vi "Periodic Tasks.vi"(8 "error in":errorcluster) -> ()   [LabVIEW 2018]
doc: "This VI runs in parallel to other tasks. It can contain as many user-defined periodic loops as you need. These can carry out PID or other sorts of timed response."
uses:
  <vilib>/Rock Robotics/WPI/Solenoid/WPI_SolenoidValue.ctl
  <vilib>/Rock Robotics/WPI/ThirdParty/Phoenix-LabVIEW/Motor Controller/Controls/CTRE_Phoenix_MotorControl_ControlMode.ctl
  <vilib>/Rock Robotics/WPI/Utilities/WPI_GetSetVariantRefNum.vi
  <vilib>/Rock Robotics/WPI/Solenoid/WPI_SolenoidSetEnum.vi
  <vilib>/Rock Robotics/WPI/ThirdParty/Phoenix-LabVIEW/Motor Controller/Get/CTRE_Phoenix_MotorController_GetQuadratureData.vi
  <vilib>/Rock Robotics/WPI/ThirdParty/Phoenix-LabVIEW/Pigeon IMU/CTRE_PigeonIMU_GetYPR.vi
  <vilib>/Rock Robotics/WPI/ThirdParty/Phoenix-LabVIEW/Pigeon IMU/CTRE_PigeonIMU_GetRawGyro.vi
  <vilib>/Rock Robotics/WPI/ThirdParty/Phoenix-LabVIEW/Pigeon IMU/CTRE_PigeonIMU_GetTempStateUpTime.vi
  <vilib>/Rock Robotics/Network Tables/NT Write Numeric Array.vi
  <vilib>/Rock Robotics/Network Tables/NT Read Number.vi
  <vilib>/addons/control/pid/pid.llb/PID Gain Schedule (DBL).vi
  <vilib>/addons/control/pid/pid.llb/PID (DBL).vi
  <vilib>/Rock Robotics/WPI/ThirdParty/Phoenix-LabVIEW/Pigeon IMU/CTRE_PigeonIMU_PigeonState.ctl
  <vilib>/addons/control/pid/NI_PID_pid.lvlib
panel:
  in  "M":dbl=0.0005
  out "X VISION":dbl=-0.020652084350585936
  out "tx":dbl=0.1304168701171875
  in  "Offset":dbl
  out "index out":i32
  in  "PID gain schedule":T1(array[cluster])=[{"PID gains"={"proportional gain (Kc)"=0.005, "integral time (Ti, min)"=0.0, "derivative time (Td, min)"=0.003}, "max value"=5.0}, {"PID gains"={"proportional gain (Kc)"=0.0105, "integral time (Ti, min)"=0.0, "derivative time (Td, min)"=0.003}, "max value"=8.0}, {"PID gains"={"proportional gain (Kc)"=0.024, "integral time (Ti, min)"=0.0, "derivative time (Td, min)"=0.0}, "max value"=12.0}, {"PID gains"={"proportional gain (Kc)"=0.02, "integral time (Ti, min)"=0.0, "derivative time (Td, min)"=0.0}, "max value"=18.0}, {"PID gains"={"proportional gain (Kc)"=0.01, "integral time (Ti, min)"=0.0, "derivative time (Td, min)"=0.0}, "max value"=25.0}] {"max value" format="%.2f"; "PID gains"."derivative time (Td, min)" format="%.3f"; "PID gains"."integral time (Ti, min)" format="%.3f"; "PID gains"."proportional gain (Kc)" format="%.3f"}
  out "tx":dbl=0.1304168701171875
  in  "Offset":dbl
  out "Left Drive Position":i32
  out "Right Drive Position":i32
  out "Right Drive Velocity":i32(graph)
  out "Left Drive Velocity":i32(graph)
  out "X VISION":dbl=-0.020652084350585936
  in  "X-Offset":dbl
  in  "PID gain schedule for vision":T1(array[cluster])=[{"PID gains"={"proportional gain (Kc)"=0.005, "integral time (Ti, min)"=0.0, "derivative time (Td, min)"=0.003}, "max value"=5.0}, {"PID gains"={"proportional gain (Kc)"=0.0105, "integral time (Ti, min)"=0.0, "derivative time (Td, min)"=0.003}, "max value"=8.0}, {"PID gains"={"proportional gain (Kc)"=0.024, "integral time (Ti, min)"=0.0, "derivative time (Td, min)"=0.0}, "max value"=12.0}, {"PID gains"={"proportional gain (Kc)"=0.02, "integral time (Ti, min)"=0.0, "derivative time (Td, min)"=0.0}, "max value"=18.0}, {"PID gains"={"proportional gain (Kc)"=0.01, "integral time (Ti, min)"=0.0, "derivative time (Td, min)"=0.0}, "max value"=25.0}] {"max value" format="%.2f"; "PID gains"."derivative time (Td, min)" format="%.3f"; "PID gains"."integral time (Ti, min)" format="%.3f"; "PID gains"."proportional gain (Kc)" format="%.3f"}
  in  "Y tracking max speed":dbl(slide)=0.7700348432055749 scale=0.0..1.0
  in  "line tracker speed":dbl=1.0
  out "C.Monitoring":bool
  out "C.Running":bool
  out "Mechanism Angle":i32
  in  "Target Distance":dbl
  in  "Target Angle":dbl
  in  "Control Type":T2(ring)
  in  "Acceleration":i32=1200
  in  "Cruise Velocity":i32=750
  in  "Shoot TIme":u32=2000
  in  "F":dbl=4.0 format="%#_13g"
  in  "D":dbl=20.0 format="%#_13g"
  in  "P":dbl=2.0
  in  "Max Reset Speed":dbl=-0.5
  in  "Max Shoot Speed":dbl=1.0
  in  "Cat Stop Position":i32=1000
  out "Mechanism Velocity":i32(graph)
  out "Mechanism Position":i32(graph)
  out "Mechanism Loop Speed":u32
  in  "D gyro":dbl
  in  "P gyro":dbl
  out "Drive Loop Speed":u32
  # "Drive By Gyro Gains"
  # "Gain schedule eqn constant for turret PID"
  # "PID COntrols"
  # "Motion Magic Controls"
  # "This limits the Y or forward speed during line following"
  # "THis ratios the x value\nset by the line follower"
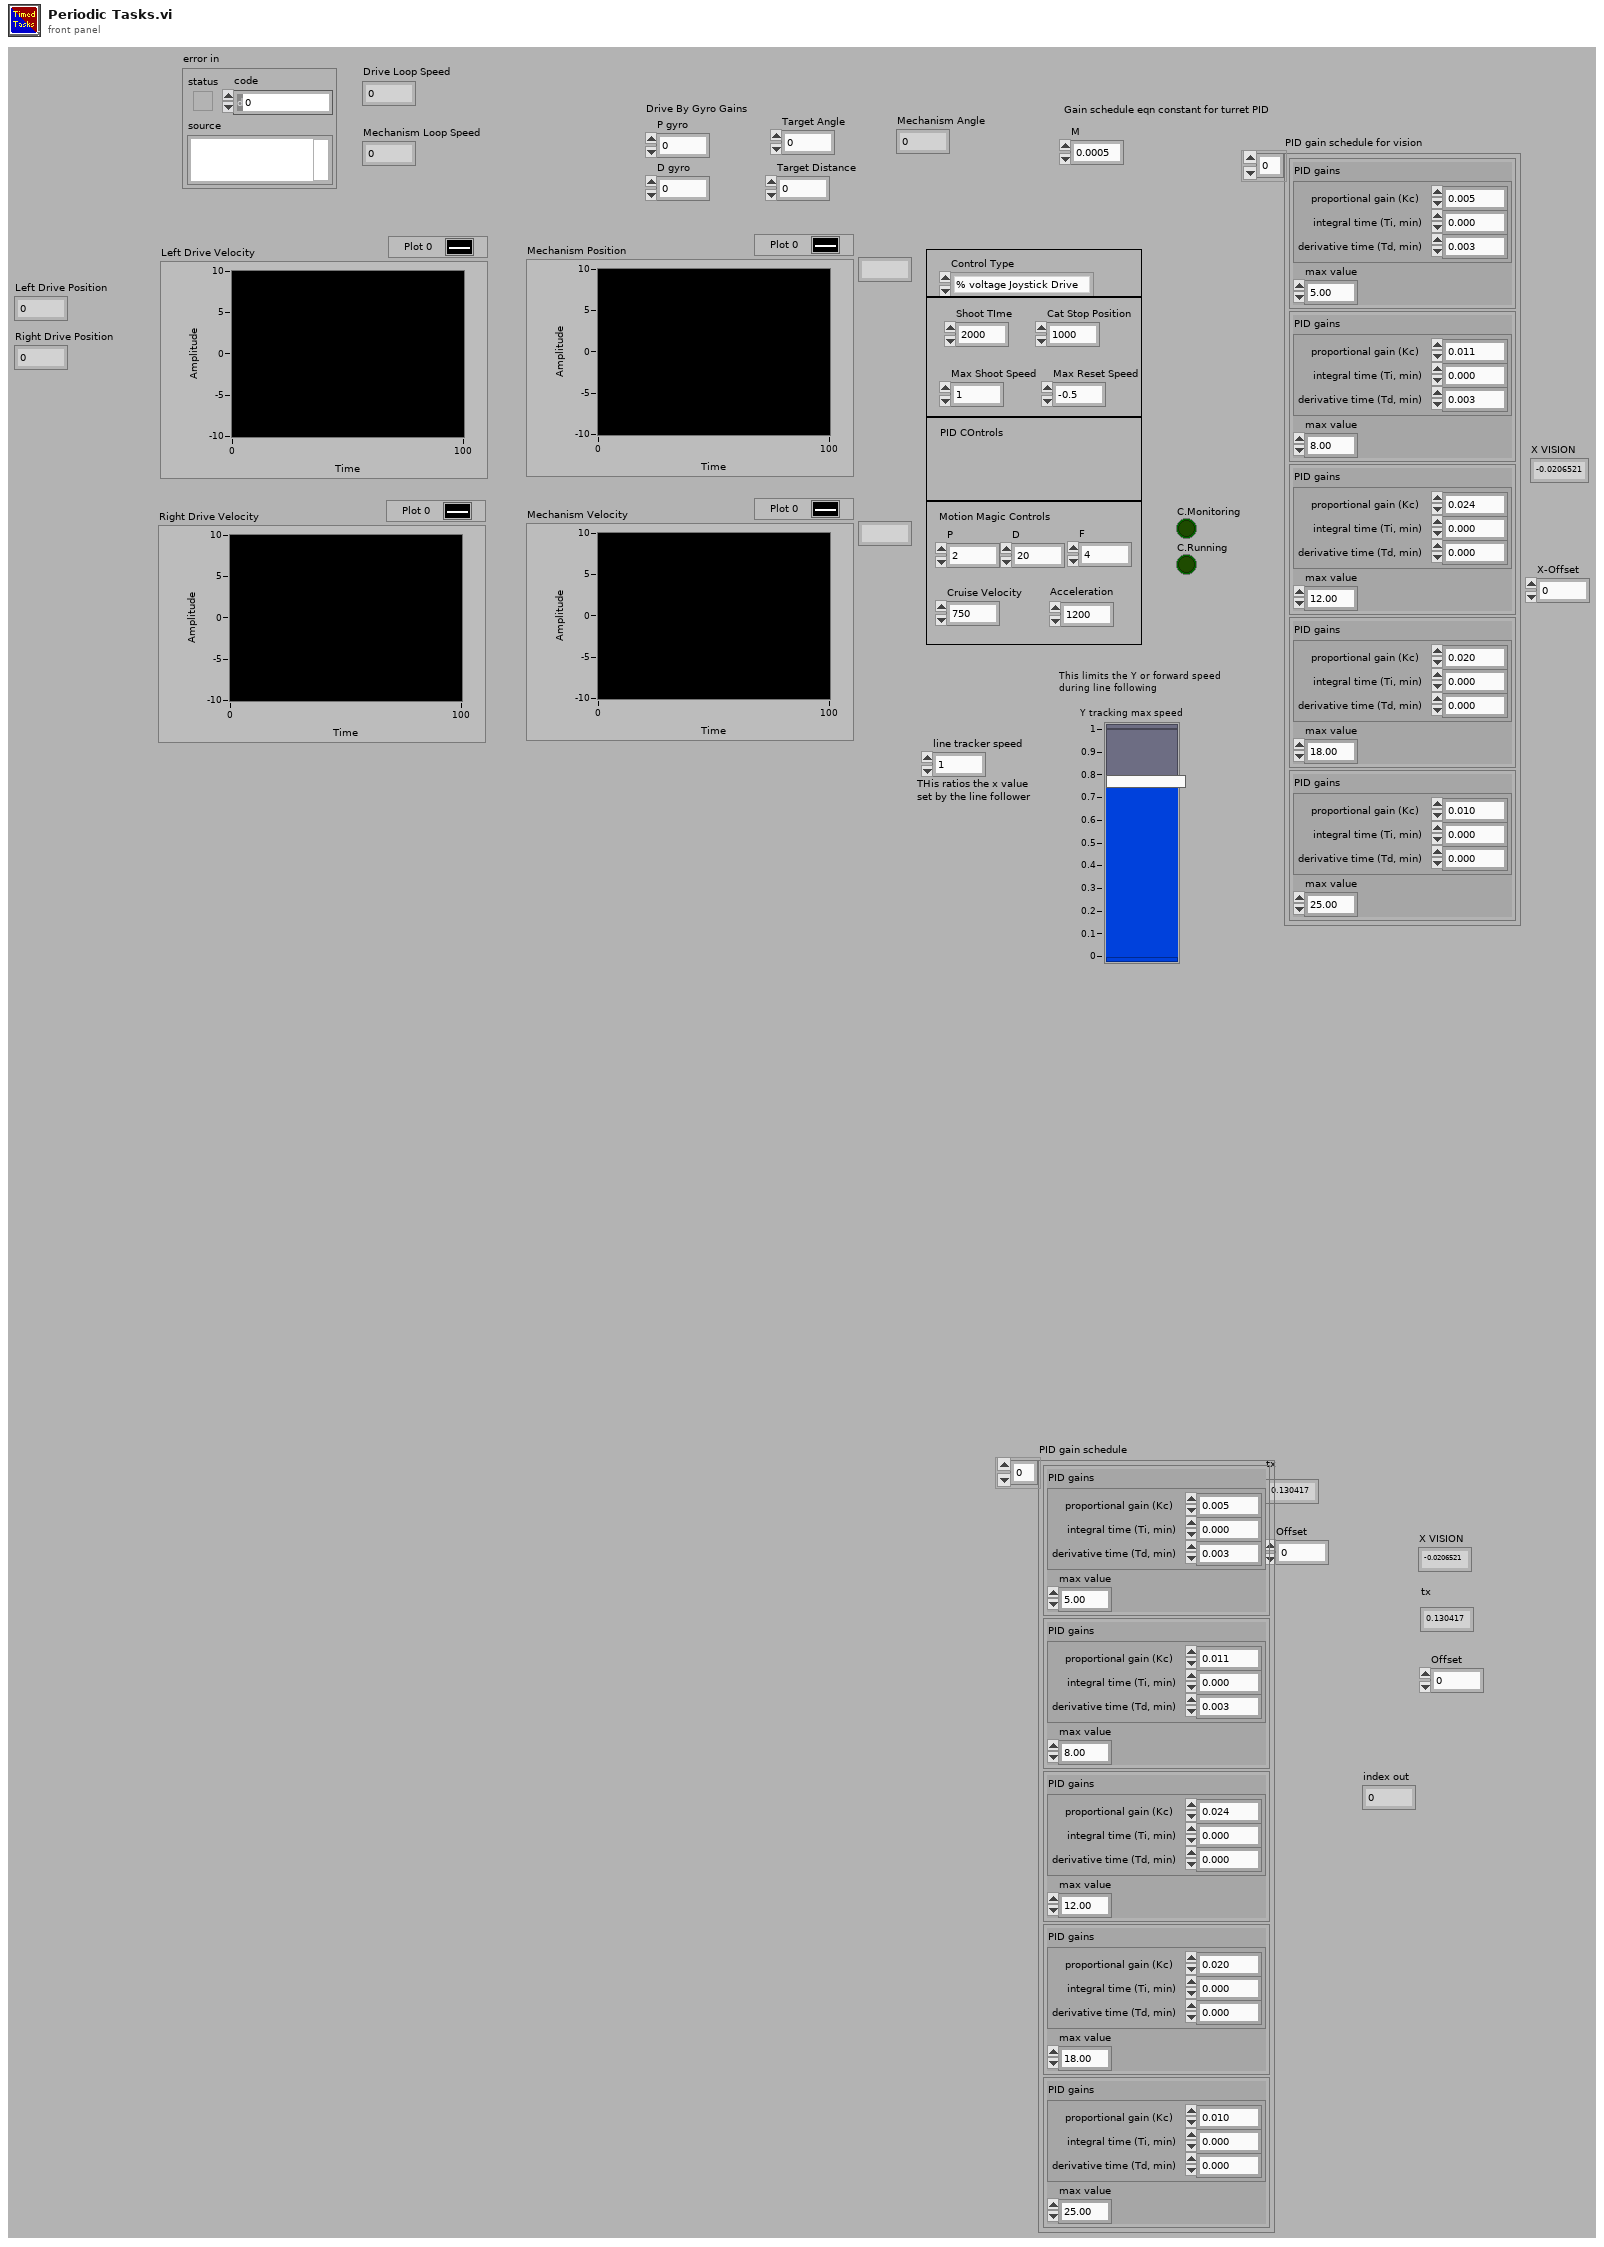
[diagram p1: front panel]
types:
  T1 = cluster{"PID gains":cluster{"proportional gain (Kc)":dbl, "integral time (Ti, min)":dbl, "derivative time (Td, min)":dbl}, "max value":dbl}[]
  T2 = enum16{"% voltage Joystick Drive", "Motion Magic Control", "PID Position Control", "Bang Bang Control"}
  T3 = typedef "WPI_DigitalInputDevRef.ctl" = cluster{"DevStatus":errorcluster, "DIO Channel":T4}
  T4 = typedef "FPGA_DIOChannel.ctl" = enum8{"DIO 0", "DIO 1", "DIO 2", "DIO 3", "DIO 4", "DIO 5", "DIO 6", "DIO 7", "DIO 8", "DIO 9", "DIO MXP 0", "DIO MXP 1", "DIO MXP 2", "DIO MXP 3", "DIO MXP 4", "DIO MXP 5", "DIO MXP 6", "DIO MXP 7", "DIO MXP 8", "DIO MXP 9", "DIO MXP 10", "DIO MXP 11", "DIO MXP 12", "DIO MXP 13", "DIO MXP 14", "DIO MXP 15", "SPI Port CS1", "SPI Port CS2", "SPI Port CS3", "SPI Port MISO", "SPI Port MOSI", "Invalid"}
  T5 = typedef "WPI_JoystickDevRef.ctl" = cluster{"Device":T6}
  T6 = typedef "WPI_JoystickDeviceEnum.ctl" = enum16{"USB 0", "USB 1", "USB 2", "USB 3", "USB 4", "USB 5"}
  T7 = typedef "CTRE_PigeonIMU_DeviceRef.ctl" = cluster{"DeviceStatus":errorcluster, "Device Number":u8, "Type":T8, "Device ID":u32, "Handle":u64, "UsageFrame":u32, "Library Path":path}
  T8 = typedef "CTRE_PigeonIMU_ConnectionType.ctl" = u32
  T9 = typedef "WPI_MotorControlDeviceRef.ctl" = cluster{"DeviceStatus":errorcluster, "Type":T10, "PWM":cluster{"PWM Channel":T11, "DeadBand":T12}, "CAN":cluster{"Device Number":u8, "SetOutput VI Ref":variant, "GetOutput VI Ref":variant, "Enable VI Ref":variant, "Disable VI Ref":variant, "Data":variant}, "Invert":bool, "DIO PWM":cluster{"PWM \"Enable\" Channel":T11, "DIOChannel":T4, "PWM Rate":dbl}}
  T10 = typedef "WPI_MotorControlType.ctl" = enum16{"PWM", "CAN", "DIO PWM"}
  T11 = typedef "FPGA_DIOPWMChannel.ctl" = enum8{"PWM 0", "PWM 1", "PWM 2", "PWM 3", "PWM 4", "PWM 5", "PWM 6", "PWM 7", "PWM 8", "PWM 9", "PWM MXP 0", "PWM MXP 1", "PWM MXP 2", "PWM MXP 3", "PWM MXP 4", "PWM MXP 5", "PWM MXP 6", "PWM MXP 7", "PWM MXP 8", "PWM MXP 9", "Invalid"}
  T12 = typedef "WPI_PWMDeadband.ctl" = cluster{"Name":string, "maxPositivePwm":i32, "minPositivePwm":i32, "centerPwm":i32, "maxNegativePwm":i32, "minNegativePwm":i32, "angularRange":u16}
  T13 = typedef "WPI_RobotDriveDevRef.ctl" = cluster{"DevStatus":errorcluster, "Motors[]":T9[], "Square Inputs":bool, "Max Output":dbl}
  T14 = enum16{"Line Following", "Drive to Vision Target", "Drive Distance to Gyro Heading", "Rotate to Gyro heading", "Drive Straight to Last Gyro heading", "Arcade Drive"}
  T15 = typedef "CTRE_PigeonIMU_PigeonState.ctl" = enum16{"NoComm", "Initializing", "Ready", "UserCalibration"}
  T16 = typedef "CTRE_PigeonIMU_CalibrationMode.ctl" = u16
  T17 = cluster{"CurrentMode":T16, "LastCalError":i32, "CalBooting?":bool, "PigeonState":T15, "UpTime":u32, "Temp. (C)":dbl, "Temp Compensation Event Count":u32, "No Motion Event Count":u32}
  T18 = cluster{"X":dbl, "Y":dbl, "Z":dbl, "Magnitude":dbl}
  T19 = enum16{"Turret Vision", "Puncher intake-shooter", "Catapult"}
  T20 = typedef "CTRE_Phoenix_MotorControl_ControlMode.ctl" = u16
  T21 = cluster{"proportional gain (Kc)":dbl, "integral time (Ti, min)":dbl, "derivative time (Td, min)":dbl}
  T22 = typedef "WPI_SolenoidDevRef.ctl" = cluster{"DevStatus":errorcluster, "Pneumatics Control Module":u8, "Forward Solenoid Channel":T23, "Reverse Solenoid Channel":T23}
  T23 = typedef "WPI_SolenoidChannel.ctl" = enum8{"Solenoid 0", "Solenoid 1", "Solenoid 2", "Solenoid 3", "Solenoid 4", "Solenoid 5", "Solenoid 6", "Solenoid 7", "Invalid"}
  T24 = typedef "WPI_CompressorDevRef.ctl" = cluster{"DevStatus":errorcluster, "Pneumatics Control Module":u8}
  T25 = typedef "WPI_SolenoidValue.ctl" = enum16{"Off", "On", "Forward", "Reverse"}
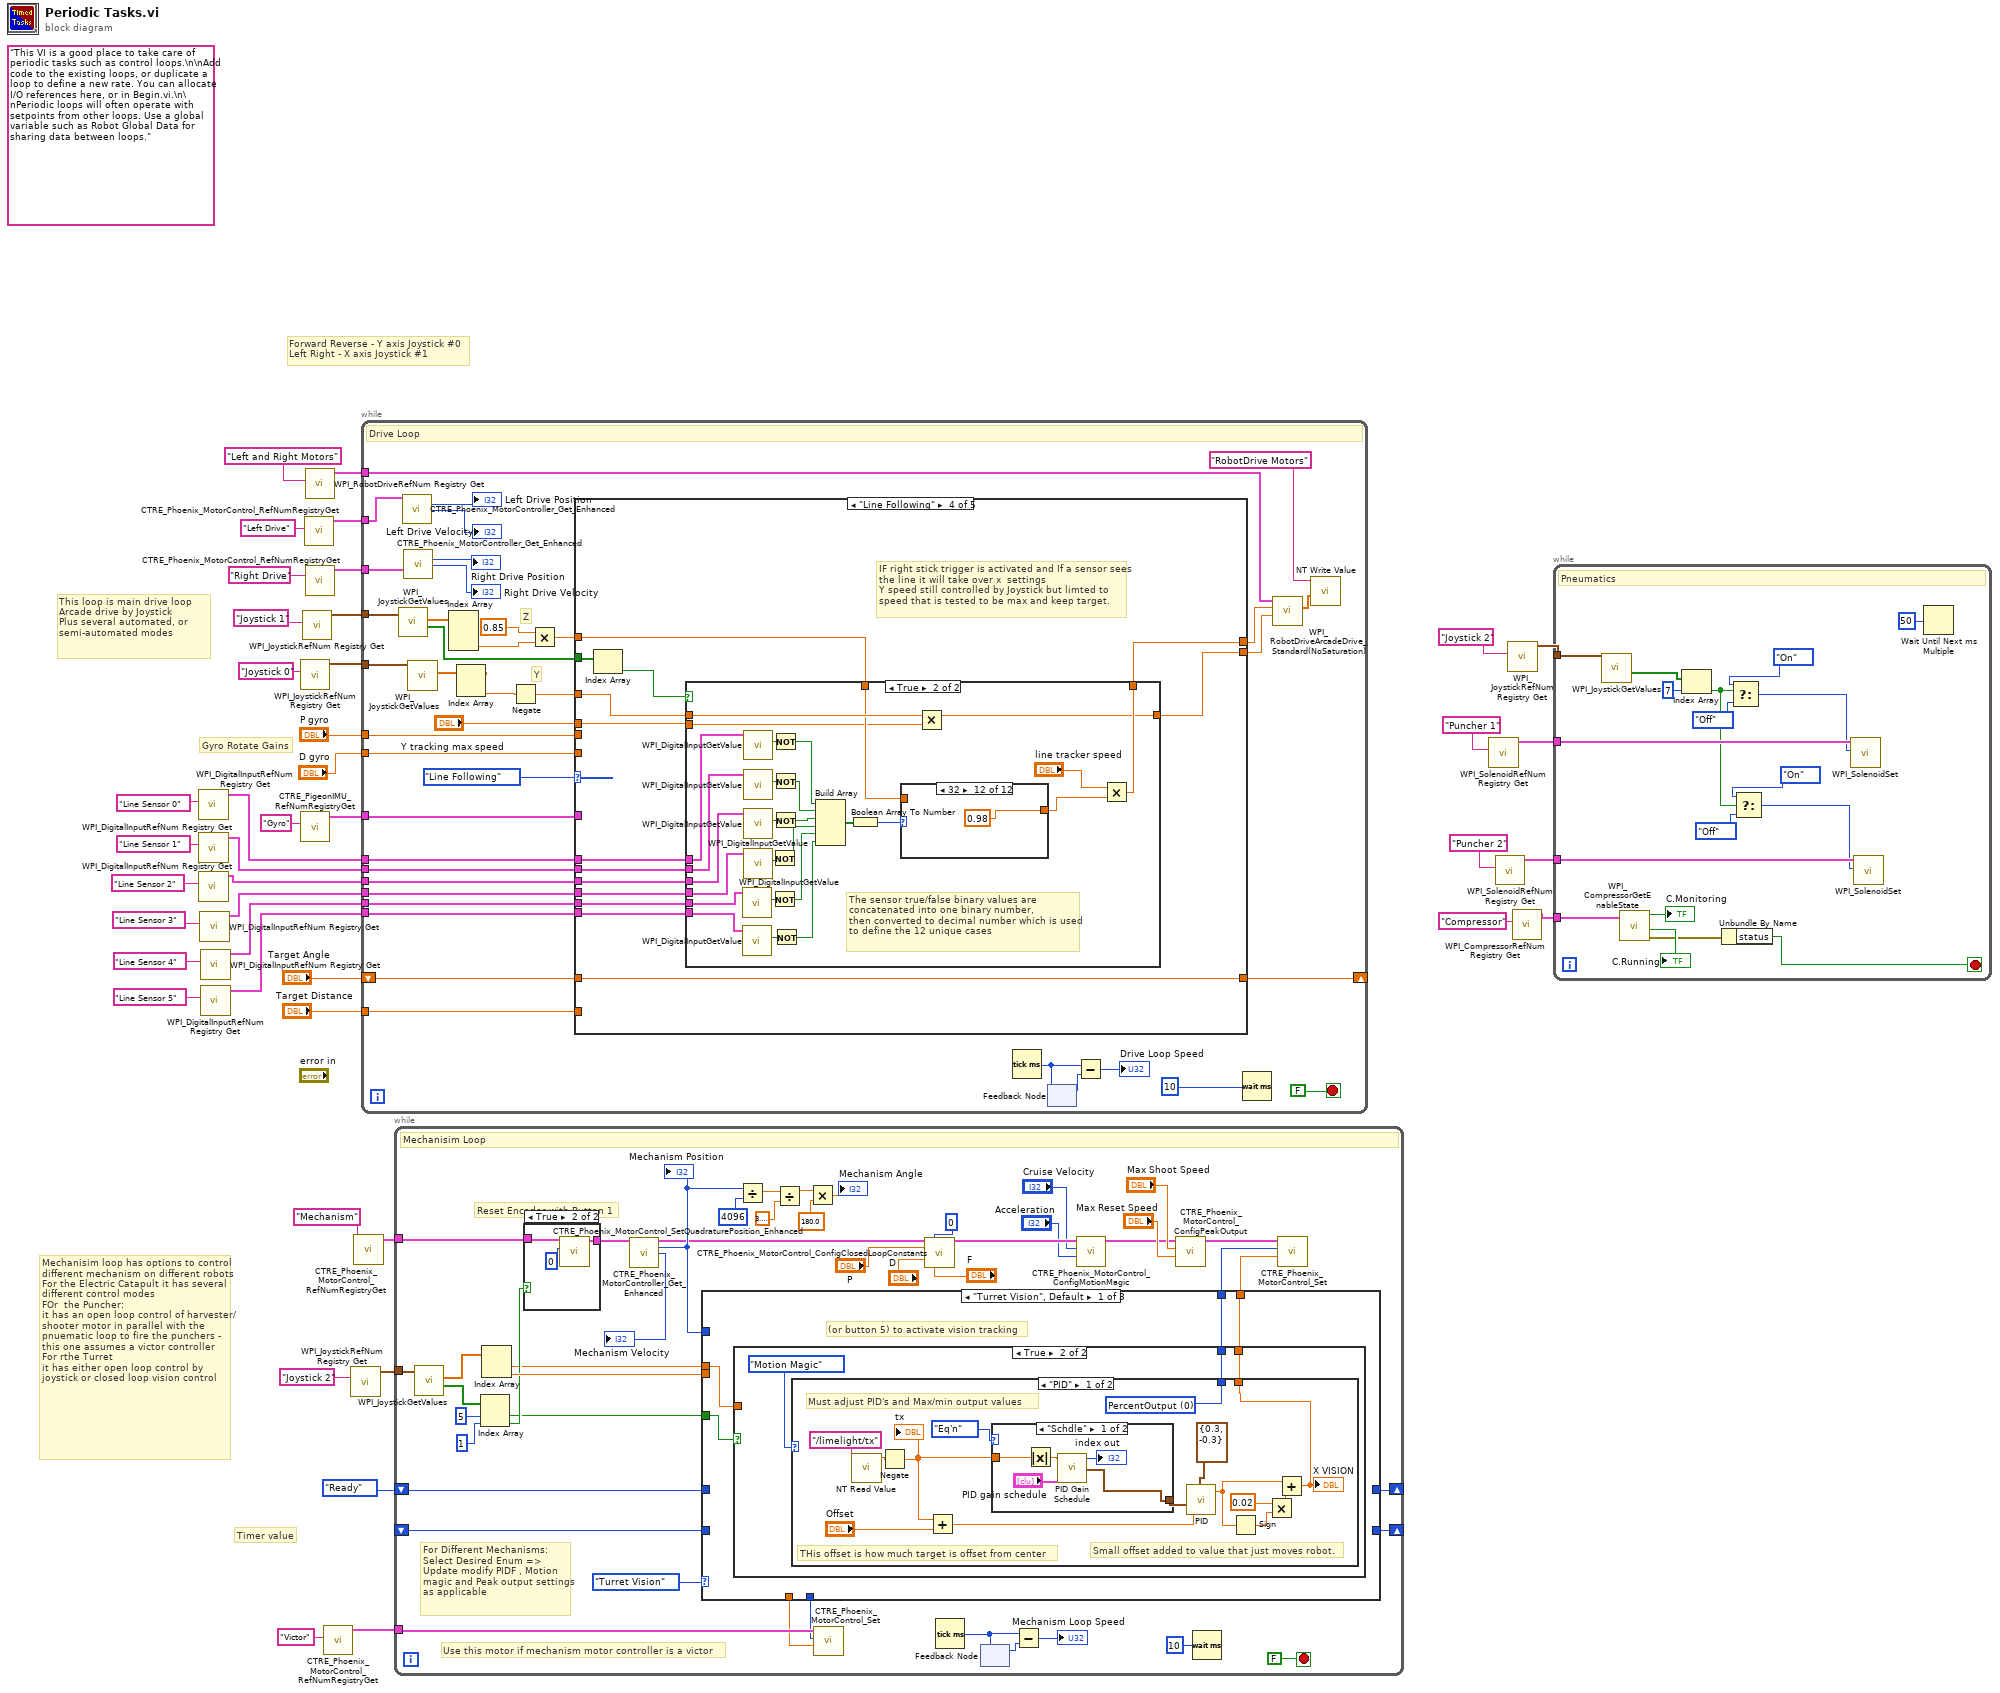
[diagram p0: block diagram]
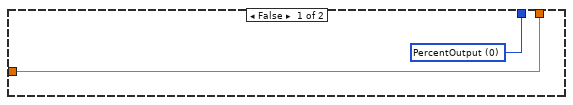
[diagram p2: hidden frame]
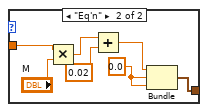
[diagram p3: hidden frame]
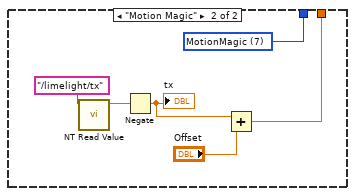
[diagram p4: hidden frame]
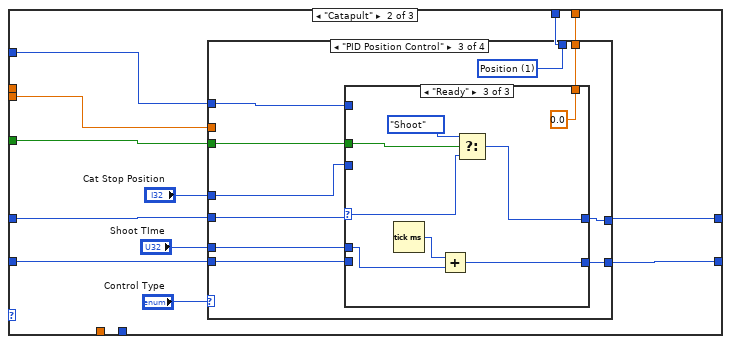
[diagram p5: hidden frame]
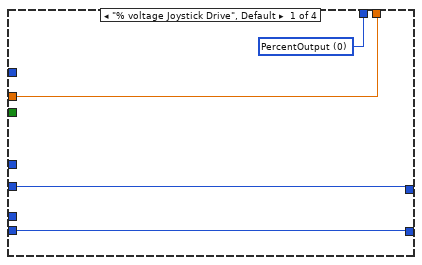
[diagram p6: hidden frame]
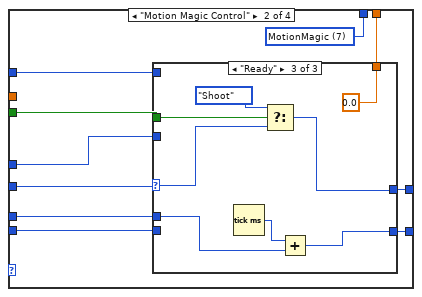
[diagram p7: hidden frame]
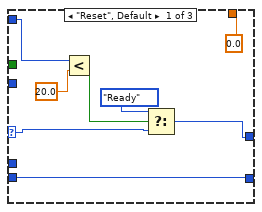
[diagram p8: hidden frame]
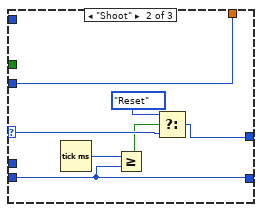
[diagram p9: hidden frame]
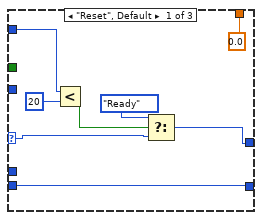
[diagram p10: hidden frame]
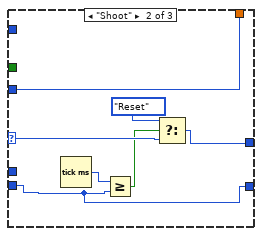
[diagram p11: hidden frame]
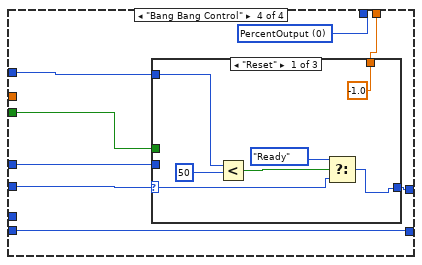
[diagram p12: hidden frame]
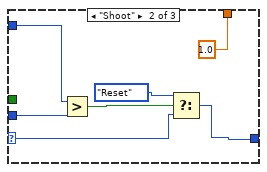
[diagram p13: hidden frame]
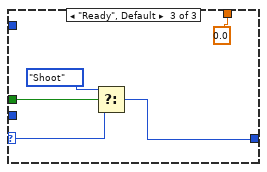
[diagram p14: hidden frame]
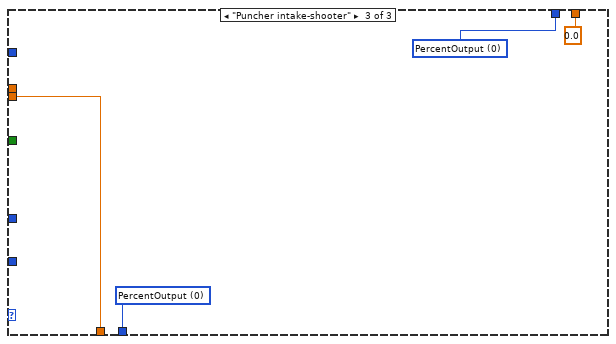
[diagram p15: hidden frame]
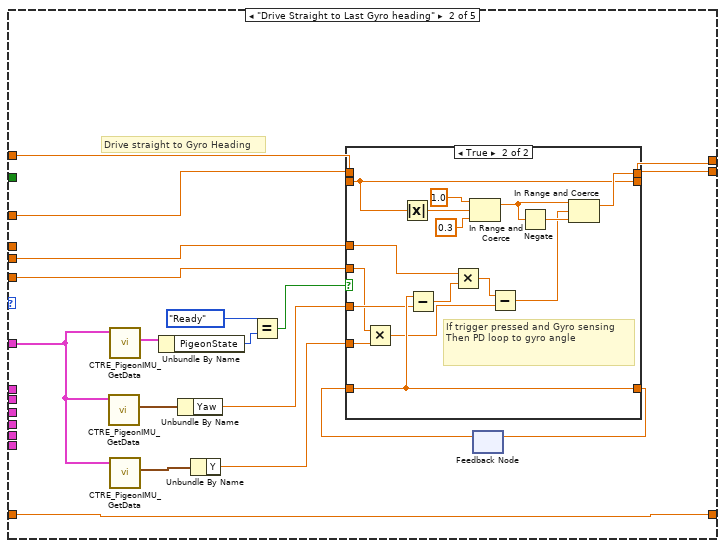
[diagram p18: hidden frame]
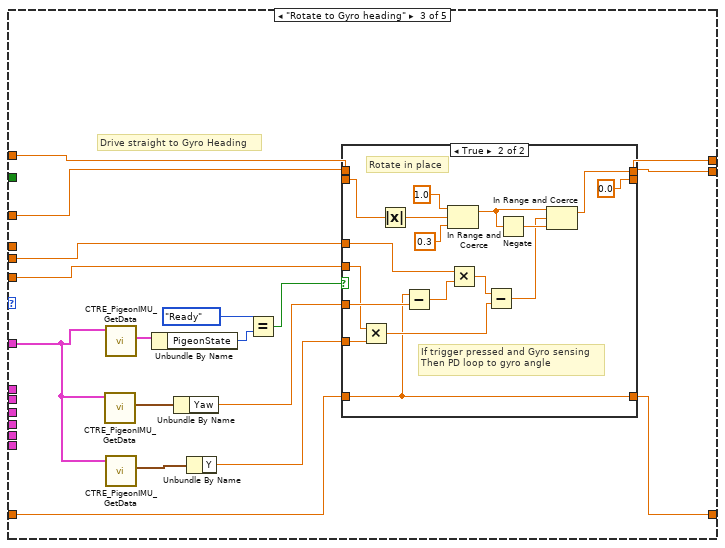
[diagram p20: hidden frame]
diagram:
  (unwired) "This VI is a good place to take care of periodic tasks such as control loops.\n\nAdd code to the existing loops, or duplicate a loop to define a new rate. You can allocate I/O references here, or in Begin.vi.\n\nPeriodic loops will often operate with setpoints from other loops. Use a global variable such as Robot Global Data for sharing data between loops."
  # "Mechanisim loop has options to control different mechanism on different robots\nFor the Electric Catapult it has several different control modes\nFOr  the Puncher:\nit has an open loop control of harvester/shooter motor in parallel with the pnuematic loop to fire the punchers - this one assumes a victor controller\nFor rthe Turret\nit has either open loop control by joystick or closed loop vision control"
  # "Timer value"
  # "This loop is main drive loop\nArcade drive by Joystick\nPlus several automated, or semi-automated modes"
  # "Gyro Rotate Gains"
  # "Forward Reverse - Y axis Joystick #0\nLeft Right - X axis Joystick #1"
  n1 = call <vilib>:"WPI_DigitalInputRefNum Registry Get.vi"("refnum name"="Line Sensor 0") -> ("DigitalInputDevRef"=w8:T3)  [unwired: 9 in, 1 out]
  n2 = call <vilib>:"WPI_DigitalInputRefNum Registry Get.vi"("refnum name"="Line Sensor 1") -> ("DigitalInputDevRef"=w7:T3)  [unwired: 9 in, 1 out]
  n3 = call <vilib>:"WPI_DigitalInputRefNum Registry Get.vi"("refnum name"="Line Sensor 2") -> ("DigitalInputDevRef"=w6:T3)  [unwired: 9 in, 1 out]
  n4 = call <vilib>:"WPI_DigitalInputRefNum Registry Get.vi"("refnum name"="Line Sensor 3") -> ("DigitalInputDevRef"=w5:T3)  [unwired: 9 in, 1 out]
  n5 = call <vilib>:"WPI_DigitalInputRefNum Registry Get.vi"("refnum name"="Line Sensor 4") -> ("DigitalInputDevRef"=w4:T3)  [unwired: 9 in, 1 out]
  n6 = call <vilib>:"WPI_DigitalInputRefNum Registry Get.vi"("refnum name"="Line Sensor 5") -> ("DigitalInputDevRef"=w3:T3)  [unwired: 9 in, 1 out]
  n7 = call <vilib>:"WPI_JoystickRefNum Registry Get.vi"("refnum name"="Joystick 0") -> ("JoystickDevRef"=w31:T5)  [unwired: 1 in, 9 out]
  n8 = call <vilib>:"CTRE_PigeonIMU_RefNumRegistryGet.vi"("refnum name"="Gyro") -> ("PigeonIMUDevRef"=w41:T7)  [unwired: 9 in, 1 out]
  n9 = call <vilib>:"WPI_JoystickRefNum Registry Get.vi"("refnum name"="Joystick 1") -> ("JoystickDevRef"=w32:T5)  [unwired: 1 in, 9 out]
  n10 = call <vilib>:"CTRE_Phoenix_MotorControl_RefNumRegistryGet.vi"("refnum name"="Left Drive") -> ("PhoenixMotorControlDevRef"=w23:T9)  [unwired: 9 in, 1 out]
  n11 = call <vilib>:"WPI_RobotDriveRefNum Registry Get.vi"("refnum name"="Left and Right Motors") -> ("RobotDriveDevRef"=w33:T13)  [unwired: 1 in, 9 out]
  n12 = call <vilib>:"CTRE_Phoenix_MotorControl_RefNumRegistryGet.vi"("refnum name"="Right Drive") -> ("PhoenixMotorControlDevRef"=w24:T9)  [unwired: 9 in, 1 out]
  n13 = call <vilib>:"CTRE_Phoenix_MotorControl_RefNumRegistryGet.vi"("refnum name"="Victor") -> ("PhoenixMotorControlDevRef"=w1:T9)  [unwired: 9 in, 1 out]
  n14 = call <vilib>:"WPI_JoystickRefNum Registry Get.vi"("refnum name"="Joystick 2") -> ("JoystickDevRef"=w30:T5)  [unwired: 1 in, 9 out]
  n15 = call <vilib>:"CTRE_Phoenix_MotorControl_RefNumRegistryGet.vi"("refnum name"="Mechanism") -> ("PhoenixMotorControlDevRef"=w29:T9)  [unwired: 9 in, 1 out]
  n16 = while {
    tunnel: w41 -> [w75]
    tunnel: "D gyro" -> [w72]
    tunnel: "P gyro" -> [w71]
    tunnel: w33 -> [w68]
    tunnel: w32 -> [w67]
    tunnel: w31 -> [w66]
    shift-right: [w63] -> _
    shift-left: "Target Angle" -> [w62]
    tunnel: "Target Distance" -> [w60]
    tunnel: w24 -> [w59]
    tunnel: w23 -> [w58]
    tunnel: w8 -> [w57]
    tunnel: w7 -> [w56]
    tunnel: w6 -> [w55]
    tunnel: w5 -> [w54]
    tunnel: w4 -> [w53]
    tunnel: w3 -> [w52]
    stop <- FALSE stop-if-true
    # "Y"
    # "Z"
    # "Drive Loop"
    n17 = call <vilib>:"WPI_JoystickGetValues.vi"("JoystickDevRef"=w67) -> ("Buttons"=w51:bool[], "Axes"=w81:dbl[])  [unwired: 6 in, 3 out]
    n18 = call-poly <vilib>:"CTRE_Phoenix_MotorController_Get_Enhanced.vi"("PhoenixMotorControlDevRef"=w58) -> ("Quadrature Position"=→"Left Drive Position":i32, "Quadrature Velocity"=→"Left Drive Velocity":i32)  [unwired: 11 in, 2 out]
    n19 = call-poly <vilib>:"CTRE_Phoenix_MotorController_Get_Enhanced.vi"("PhoenixMotorControlDevRef"=w59) -> ("Quadrature Position"=→"Right Drive Position":i32, "Quadrature Velocity"=→"Right Drive Velocity":i32)  [unwired: 11 in, 2 out]
    n20 = call <vilib>:"WPI_JoystickGetValues.vi"("JoystickDevRef"=w66) -> ("Axes"=w70:dbl[])  [unwired: 6 in, 4 out]
    n21 = Index Array(array=w81) -> (element #3=w65:dbl)  [unwired: 3 in, 2 out]
    n22 = Index Array(array=w70) -> (element #2=w48:dbl)  [unwired: 2 in, 1 out]
    n23 = Negate(x=w48) -> (-x=w50:dbl)
    n24 = Multiply(x=0.85, y=w65) -> (x*y=w61:dbl)
    n25 = case shown="\"Line Following\"" T14."Line Following" {
      tunnel: w50 -> [w85 w104 w129 w162 w219]
      tunnel: w61 -> [w86 w103 w128 w163 w216]
      tunnel: w75 -> [_ w98 w132 _ _]
      tunnel: [w86 w93 w126 w168 w223] -> w74
      tunnel: [w85 w92 w127 w164 w221] -> w73
      tunnel: w72 -> [_ w89 w131 _ _]
      tunnel: w71 -> [_ w88 w130 _ _]
      tunnel: w62 -> [w84 w87 w125 w167 w222]
      tunnel: [w84 w87 w124 w167 w222] -> w63
      tunnel: w60 -> [_ _ _ _ _]
      tunnel: w57 -> [_ _ _ w169 _]
      tunnel: w56 -> [_ _ _ w170 _]
      tunnel: w55 -> [_ _ _ w171 _]
      tunnel: w54 -> [_ _ _ w172 _]
      tunnel: w53 -> [_ _ _ w173 _]
      tunnel: w52 -> [_ _ _ w174 _]
      tunnel: w51 -> [_ _ _ w166 w218]
      tunnel: "Y tracking max speed" -> [_ _ _ w161 w220]
      frame "Arcade Drive", Default {
      }
      frame "Drive Straight to Last Gyro heading" {
        # "Drive straight to Gyro Heading"
        n26 = call-poly <vilib>:"CTRE_PigeonIMU_GetData.vi"("PigeonIMUDevRef"=w98) -> ("Yaw Pitch Roll"=w96:cluster{"Yaw":dbl, "Pitch":dbl, "Roll":dbl})  [unwired: 8 in, 2 out]
        n27 = call-poly <vilib>:"CTRE_PigeonIMU_GetData.vi"("PigeonIMUDevRef"=w98) -> ("Temp/State/UpTime"=w102:T17)  [unwired: 8 in, 2 out]
        n28 = call-poly <vilib>:"CTRE_PigeonIMU_GetData.vi"("PigeonIMUDevRef"=w98) -> ("Gyro DPS"=w97:T18)  [unwired: 8 in, 2 out]
        n29 = Unbundle By Name(w102) -> ("PigeonState"=w101:T15)
        n30 = Unbundle By Name(w96) -> ("Yaw"=w95:dbl)
        n31 = Unbundle By Name(w97) -> ("Y"=w94:dbl)
        n32 = Equal?(x=CTRE_PigeonIMU_PigeonState."Ready", y=w101) -> (x = y?=w99:bool)
        n33 = feedback #1() -> (w90:dbl)  [unwired: 1 in]
        n34 = case shown="True" w99 {
          tunnel: w104 -> [w106 w108]
          tunnel: w103 -> [w107 _]
          tunnel: w95 -> [w105 w117]
          tunnel: w94 -> [_ w113]
          tunnel: [w105 w118] -> w91
          tunnel: [w107 w109] -> w93
          tunnel: [w106 w108] -> w92
          tunnel: w90 -> [_ w118]
          tunnel: w89 -> [_ w114]
          tunnel: w88 -> [_ w116]
          frame False {
          }
          frame True {
            # "If trigger pressed and Gyro sensing\nThen PD loop to gyro angle"
            n35 = Multiply(x=w114, y=w113) -> (x*y=w111:dbl)
            n36 = Absolute Value(x=w108) -> (abs(x)=w121:dbl)
            n37 = Subtract(x=w118, y=w117) -> (x-y=w115:dbl)
            n38 = Multiply(x=w116, y=w115) -> (x*y=w112:dbl)
            n39 = In Range and Coerce(upper limit=1.0, x=w121, lower limit=0.3) -> (coerced(x)=w119:dbl)  [unwired: 1 out]
            n40 = Subtract(x=w112, y=w111) -> (x-y=w110:dbl)
            n41 = Negate(x=w119) -> (-x=w120:dbl)
            n42 = In Range and Coerce(upper limit=w119, x=w110, lower limit=w120) -> (coerced(x)=w109:dbl)  [unwired: 1 out]
          }
        }
        n43 = feedback-in #1(w91) -> ()
      }
      frame "Rotate to Gyro heading" {
        # "Drive straight to Gyro Heading"
        n44 = call-poly <vilib>:"CTRE_PigeonIMU_GetData.vi"("PigeonIMUDevRef"=w132) -> ("Yaw Pitch Roll"=w135:cluster{"Yaw":dbl, "Pitch":dbl, "Roll":dbl})  [unwired: 8 in, 2 out]
        n45 = call-poly <vilib>:"CTRE_PigeonIMU_GetData.vi"("PigeonIMUDevRef"=w132) -> ("Temp/State/UpTime"=w140:T17)  [unwired: 8 in, 2 out]
        n46 = call-poly <vilib>:"CTRE_PigeonIMU_GetData.vi"("PigeonIMUDevRef"=w132) -> ("Gyro DPS"=w136:T18)  [unwired: 8 in, 2 out]
        n47 = Unbundle By Name(w140) -> ("PigeonState"=w139:T15)
        n48 = Unbundle By Name(w135) -> ("Yaw"=w134:dbl)
        n49 = Unbundle By Name(w136) -> ("Y"=w133:dbl)
        n50 = Equal?(x=CTRE_PigeonIMU_PigeonState."Ready", y=w139) -> (x = y?=w137:bool)
        n51 = case shown="True" w137 {
          tunnel: w129 -> [w142 w146]
          tunnel: w128 -> [w143 _]
          tunnel: w134 -> [_ w155]
          tunnel: w133 -> [_ w151]
          tunnel: [w143 w147] -> w126
          tunnel: [w142 0.0 ("upper limit")] -> w127
          tunnel: w131 -> [_ w152]
          tunnel: w130 -> [_ w154]
          tunnel: w125 -> [w141 w144]
          tunnel: [w141 w144] -> w124
          frame False {
          }
          frame True {
            # "Rotate in place"
            # "If trigger pressed and Gyro sensing\nThen PD loop to gyro angle"
            n52 = Multiply(x=w152, y=w151) -> (x*y=w149:dbl)
            n53 = Absolute Value(x=w146) -> (abs(x)=w158:dbl)
            n54 = Subtract(x=w144, y=w155) -> (x-y=w153:dbl)
            n55 = In Range and Coerce(upper limit=1.0, x=w158, lower limit=0.3) -> (coerced(x)=w156:dbl)  [unwired: 1 out]
            n56 = Multiply(x=w154, y=w153) -> (x*y=w150:dbl)
            n57 = Subtract(x=w150, y=w149) -> (x-y=w148:dbl)
            n58 = Negate(x=w156) -> (-x=w157:dbl)
            n59 = In Range and Coerce(upper limit=w156, x=w148, lower limit=w157) -> (coerced(x)=w147:dbl)  [unwired: 1 out]
          }
        }
      }
      frame "Line Following" {
        # "IF right stick trigger is activated and If a sensor sees the line it will take over x  settings\nY speed still controlled by Joystick but limted to speed that is tested to be max and keep target."
        n60 = Index Array(array=w166) -> (element=w165:bool)  [unwired: 1 in]
        n61 = case shown="True" w165 {
          tunnel: w174 -> [_ w187]
          tunnel: w173 -> [_ w186]
          tunnel: w172 -> [_ w185]
          tunnel: w171 -> [_ w184]
          tunnel: w170 -> [_ w183]
          tunnel: w169 -> [_ w182]
          tunnel: [w175 w181] -> w168
          tunnel: w162 -> [w176 w180]
          tunnel: [w176 w179] -> w164
          tunnel: w163 -> [w175 w178]
          tunnel: w161 -> [_ w177]
          frame False {
          }
          frame True {
            # "The sensor true/false binary values are concatenated into one binary number,\nthen converted to decimal number which is used to define the 12 unique cases"
            n62 = call <vilib>:"WPI_DigitalInputGetValue.vi"("DigitalInputDevRef"=w186) -> ("Value"=w201:bool)  [unwired: 8 in, 2 out]
            n63 = call <vilib>:"WPI_DigitalInputGetValue.vi"("DigitalInputDevRef"=w187) -> ("Value"=w200:bool)  [unwired: 8 in, 2 out]
            n64 = call <vilib>:"WPI_DigitalInputGetValue.vi"("DigitalInputDevRef"=w182) -> ("Value"=w199:bool)  [unwired: 8 in, 2 out]
            n65 = call <vilib>:"WPI_DigitalInputGetValue.vi"("DigitalInputDevRef"=w183) -> ("Value"=w198:bool)  [unwired: 8 in, 2 out]
            n66 = call <vilib>:"WPI_DigitalInputGetValue.vi"("DigitalInputDevRef"=w184) -> ("Value"=w202:bool)  [unwired: 8 in, 2 out]
            n67 = call <vilib>:"WPI_DigitalInputGetValue.vi"("DigitalInputDevRef"=w185) -> ("Value"=w197:bool)  [unwired: 8 in, 2 out]
            n68 = Not(x=w197) -> (.not. x?=w193:bool)
            n69 = Not(x=w201) -> (.not. x?=w192:bool)
            n70 = Not(x=w199) -> (.not. x?=w196:bool)
            n71 = Not(x=w198) -> (.not. x?=w195:bool)
            n72 = Not(x=w202) -> (.not. x?=w194:bool)
            n73 = Not(x=w200) -> (.not. x?=w191:bool)
            n74 = Build Array(w196, w195, w194, w193, w192, w191) -> (w203:bool[])
            n75 = Boolean Array To Number(Boolean array=w203) -> (number=w188:u32)
            n76 = case shown="32" w188 {
              tunnel: [w204 -0.98 ("X") -0.79 ("X") -0.6 ("X") -0.525 ("X") -0.45 ("X") 0.0 ("X") 0.45 ("X") 0.525 ("X") 0.6 ("X") 0.79 ("X") 0.98 ("X")] -> w189
              tunnel: w178 -> [w204 _ _ _ _ _ _ _ _ _ _ _]
              frame 0, Default {
                # "No target seen\nleave to joystick"
              }
              frame 1 {
              }
              frame 3 {
              }
              frame 2 {
              }
              frame 6 {
              }
              frame 4 {
              }
              frame 12 {
              }
              frame 8 {
              }
              frame 24 {
              }
              frame 16 {
              }
              frame 48 {
              }
              frame 32 {
              }
            }
            n77 = Multiply(x=w180, y=w177) -> (x*y=w179:dbl)
            n78 = Multiply(x="line tracker speed", y=w189) -> (x*y=w181:dbl)
          }
        }
      }
      frame "Drive to Vision Target" {
        # "Activate Vision by pressing Joystick 1 Trigger"
        n79 = Index Array(array=w218) -> (element=w217:bool)  [unwired: 1 in]
        n80 = Multiply(x=w219, y=w220) -> (x*y=w221:dbl)
        n81 = case shown="True" w217 {
          tunnel: [w224 w225] -> w223
          tunnel: w216 -> [w224 _]
          frame False {
          }
          frame True {
            n82 = call "X Vision.vi"("PID gain schedule for vision"="PID gain schedule for vision", "Offset"="X-Offset") -> ("X VISION"=w225:dbl)  [unwired: 4 in]
            "X VISION" <- w225
          }
        }
      }
    }
    n83 = Tick Count (ms)() -> (millisecond timer value=w78:u32)
    n84 = feedback-in #2(w78) -> ()
    n85 = feedback #2() -> (w77:u32)  [unwired: 1 in]
    n86 = Subtract(x=w78, y=w77) -> (x-y=→"Drive Loop Speed":u32)
    n87 = Wait (ms)(milliseconds to wait=u32 10) -> ()  [unwired: 1 out]
    n88 = call <vilib>:"WPI_RobotDriveArcadeDrive_Standard(NoSaturation).vi"("Y axis value"=w73, "X axis value"=w74, "RobotDriveDevRef"=w68) -> ("Motor Values"=w80:dbl[])  [unwired: 1 in, 7 out]
    n89 = call-poly <vilib>:"NT Write Value.vi"("Numeric Array"=w80, "Name"="RobotDrive Motors") -> ()  [unwired: 9 in, 1 out]
  }
  n90 = while {
    shift-right: [w260] -> _
    shift-left: enum16{"Reset", "Shoot", "Ready"}."Ready" -> [w259]
    shift-right: [w258] -> _
    shift-left: _ -> [w257]
    tunnel: w30 -> [w255]
    tunnel: w29 -> [w256]
    tunnel: w1 -> [w231]
    stop <- FALSE stop-if-true
    # "Use this motor if mechanism motor controller is a victor"
    # "For Different Mechanisms:\nSelect Desired Enum =>\nUpdate modify PIDF , Motion magic and Peak output settings as applicable"
    # "Reset Encoder with Button 1"
    # "Mechanisim Loop"
    n91 = call <vilib>:"WPI_JoystickGetValues.vi"("JoystickDevRef"=w255) -> ("Buttons"=w267:bool[], "Axes"=w268:dbl[])  [unwired: 6 in, 3 out]
    n92 = Index Array(array=w267, index #1=5 ("index"), index #2=1 ("index")) -> (element #1=w261:bool, element #2=w263:bool)
    n93 = Index Array(array=w268) -> (element #1=w228:dbl, element #2=w266:dbl)  [unwired: 2 in]
    n94 = case shown="True" w263 {
      tunnel: [w428 w430] -> w262
      tunnel: w256 -> [w428 w429]
      frame False {
      }
      frame True {
        n95 = call <vilib>:"CTRE_Phoenix_MotorControl_SetQuadraturePosition_Enhanced.vi"("New Position"=0, "PhoenixMotorControlDevRef"=w429) -> ("PhoenixMotorControlDevRef"=w430:T9)  [unwired: 8 in, 1 out]
      }
    }
    n96 = call-poly <vilib>:"CTRE_Phoenix_MotorController_Get_Enhanced.vi"("PhoenixMotorControlDevRef"=w262) -> ("PhoenixMotorControlDevRef"=w250:T9, "Quadrature Position"=w251:i32, "Quadrature Velocity"=→"Mechanism Velocity":i32)  [unwired: 11 in, 1 out]
    "Mechanism Position" <- w251
    n97 = case shown="\"Turret Vision\", Default" T19."Turret Vision" {
      tunnel: w266 -> [_ w326 w424]
      tunnel: w261 -> [w277 w325 _]
      tunnel: [_ w324 _] -> w260
      tunnel: w259 -> [_ w323 _]
      tunnel: [_ w322 _] -> w258
      tunnel: w257 -> [_ w321 _]
      tunnel: [w276 w319 w427] -> w253
      tunnel: [w275 w318 0.0 ("Bang-Bang Cat Speed")] -> w252
      tunnel: w251 -> [_ w317 _]
      tunnel: [_ _ w425] -> w230
      tunnel: [_ _ w424] -> w229
      tunnel: w228 -> [w274 _ _]
      frame "Turret Vision", Default {
        # "(or button 5) to activate vision tracking"
        n98 = case shown="True" w277 {
          tunnel: [w279 w282] -> w276
          tunnel: w274 -> [w278 _]
          tunnel: [w278 w281] -> w275
          frame False {
            w279 = T20 0 items=["PercentOutput"=0, "Position"=1, "Velocity"=2, "Current"=3, "Follower"=5, "MotionProfile"=6, "MotionMagic"=7, "MotionProfileArc"=10, "Disabled"=15] ("Control Mode")
          }
          frame True {
            n99 = case shown="\"PID\"" enum16{"Motion Magic", "PID"}."Motion Magic" {
              tunnel: [w296 w314] -> w282
              tunnel: [w283 w309] -> w281
              frame "PID" {
                w296 = T20 0 items=["PercentOutput"=0, "Position"=1, "Velocity"=2, "Current"=3, "Follower"=5, "MotionProfile"=6, "MotionMagic"=7, "MotionProfileArc"=10, "Disabled"=15] ("Control Mode")
                # "Must adjust PID's and Max/min output values"
                # "THis offset is how much target is offset from center"
                # "Small offset added to value that just moves robot."
                n100 = call-poly <vilib>:"NT Read Value.vi"("Name"="/limelight/tx") -> ("Numeric"=w294:dbl)  [unwired: 9 in, 1 out]
                n101 = Negate(x=w294) -> (-x=w287:dbl)
                "tx" <- w287
                n102 = Add(x=w287, y="Offset") -> (x+y=w288:dbl)
                n103 = case shown="\"Schdle\"" enum16{"Eq'n", "Schdle"}."Eq'n" {
                  tunnel: w287 -> [w298 w308]
                  tunnel: [w297 w302] -> w284
                  frame "Schdle" {
                    n104 = Absolute Value(x=w298) -> (abs(x)=w301:dbl)
                    n105 = call-poly <vilib>:"PID Gain Schedule.vi"("PID gain schedule"="PID gain schedule", "gain scheduling value"=w301) -> ("PID gains out"=w297:T21, "index out"=→"index out":i32)  [unwired: 2 in]
                  }
                  frame "Eq'n" {
                    w303 = 0.0
                    n106 = Multiply(x=w308, y="M") -> (x*y=w306:dbl)
                    n107 = Add(x=w306, y=0.02) -> (x+y=w304:dbl)
                    n108 = Bundle(w304, w303, w303) -> (w302:cluster{dbl, dbl, dbl})  [unwired: 1 in]
                  }
                }
                n109 = call-poly <vilib>:"PID.vi"("output range"=cluster{"output high":dbl, "output low":dbl} {"output high"=0.3, "output low"=-0.3}, "PID gains"=w284, "process variable"=w288) -> ("output"=w292:dbl)  [unwired: 7 in, 1 out]
                n110 = Sign(1:w292) -> (0:w291:dbl)
                n111 = Multiply(x=0.02, y=w291) -> (x*y=w289:dbl)
                n112 = Add(x=w292, y=w289) -> (x+y=w283:dbl)
                "X VISION" <- w283
              }
              frame "Motion Magic" {
                w314 = T20 7 items=["PercentOutput"=0, "Position"=1, "Velocity"=2, "Current"=3, "Follower"=5, "MotionProfile"=6, "MotionMagic"=7, "MotionProfileArc"=10, "Disabled"=15] ("Control Mode")
                n113 = call-poly <vilib>:"NT Read Value.vi"("Name"="/limelight/tx") -> ("Numeric"=w312:dbl)  [unwired: 9 in, 1 out]
                n114 = Negate(x=w312) -> (-x=w311:dbl)
                "tx" <- w311
                n115 = Add(x=w311, y="Offset") -> (x+y=w309:dbl)
              }
            }
          }
        }
      }
      frame "Catapult" {
        n116 = case shown="\"PID Position Control\"" "Control Type" {
          tunnel: w326 -> [w329 _ _ _]
          tunnel: [w330 w339 w370 w404] -> w319
          tunnel: [w329 w338 w369 w400] -> w318
          tunnel: w323 -> [w328 w336 w372 w403]
          tunnel: [w328 w340 w373 w402] -> w324
          tunnel: w325 -> [_ w335 w371 w401]
          tunnel: w317 -> [_ w337 w367 w399]
          tunnel: "Cat Stop Position" -> [_ w334 w368 w398]
          tunnel: "Shoot TIme" -> [_ w332 w366 _]
          tunnel: [w327 w333 w365 w397] -> w322
          tunnel: w321 -> [w327 w331 w364 w397]
          frame "% voltage Joystick Drive", Default {
            w330 = T20 0 items=["PercentOutput"=0, "Position"=1, "Velocity"=2, "Current"=3, "Follower"=5, "MotionProfile"=6, "MotionMagic"=7, "MotionProfileArc"=10, "Disabled"=15] ("Control Mode")
          }
          frame "Motion Magic Control" {
            w339 = T20 7 items=["PercentOutput"=0, "Position"=1, "Velocity"=2, "Current"=3, "Follower"=5, "MotionProfile"=6, "MotionMagic"=7, "MotionProfileArc"=10, "Disabled"=15] ("Control Mode")
            n117 = case shown="\"Ready\"" w336 {
              selector: w336 -> [w345 w353 w361]
              tunnel: [w342 w352 w362] -> w340
              tunnel: w335 -> [_ _ w360]
              tunnel: [0.0 ("Cat Stop Position") w355 0.0] -> w338
              tunnel: w334 -> [_ w355 _]
              tunnel: w337 -> [w343 _ _]
              tunnel: w332 -> [_ _ w357]
              tunnel: [w341 w349 w356] -> w333
              tunnel: w331 -> [w341 w349 _]
              frame "Reset", Default {
                n118 = Less?(x=w343, y=20.0) -> (x < y?=w346:bool)
                n119 = Select(t=enum16{"Reset", "Shoot", "Ready"}."Ready", s=w346, f=w345) -> (s? t:f=w342:enum16{"Reset", "Shoot", "Ready"})
              }
              frame "Shoot" {
                n120 = Tick Count (ms)() -> (millisecond timer value=w351:u32)
                n121 = Greater Or Equal?(x=w351, y=w349) -> (x >= y?=w350:bool)
                n122 = Select(t=enum16{"Reset", "Shoot", "Ready"}."Reset", s=w350, f=w353) -> (s? t:f=w352:enum16{"Reset", "Shoot", "Ready"})
              }
              frame "Ready" {
                n123 = Tick Count (ms)() -> (millisecond timer value=w358:u32)
                n124 = Select(t=enum16{"Reset", "Shoot", "Ready"}."Shoot", s=w360, f=w361) -> (s? t:f=w362:enum16{"Reset", "Shoot", "Ready"})
                n125 = Add(x=w358, y=w357) -> (x+y=w356:u32)
              }
            }
          }
          frame "PID Position Control" {
            w370 = T20 1 items=["PercentOutput"=0, "Position"=1, "Velocity"=2, "Current"=3, "Follower"=5, "MotionProfile"=6, "MotionMagic"=7, "MotionProfileArc"=10, "Disabled"=15] ("Control Mode")
            n126 = case shown="\"Ready\"" w372 {
              selector: w372 -> [w378 w386 w394]
              tunnel: [w377 w385 w395] -> w373
              tunnel: w371 -> [_ _ w393]
              tunnel: [0.0 ("Cat Stop Position") w388 0.0] -> w369
              tunnel: w368 -> [_ w388 _]
              tunnel: w367 -> [w376 _ _]
              tunnel: w366 -> [_ _ w390]
              tunnel: [w374 w382 w389] -> w365
              tunnel: w364 -> [w374 w382 _]
              frame "Reset", Default {
                n127 = Less?(x=w376, y=20) -> (x < y?=w379:bool)
                n128 = Select(t=enum16{"Reset", "Shoot", "Ready"}."Ready", s=w379, f=w378) -> (s? t:f=w377:enum16{"Reset", "Shoot", "Ready"})
              }
              frame "Shoot" {
                n129 = Tick Count (ms)() -> (millisecond timer value=w384:u32)
                n130 = Greater Or Equal?(x=w384, y=w382) -> (x >= y?=w383:bool)
                n131 = Select(t=enum16{"Reset", "Shoot", "Ready"}."Reset", s=w383, f=w386) -> (s? t:f=w385:enum16{"Reset", "Shoot", "Ready"})
              }
              frame "Ready" {
                n132 = Tick Count (ms)() -> (millisecond timer value=w391:u32)
                n133 = Add(x=w391, y=w390) -> (x+y=w389:u32)
                n134 = Select(t=enum16{"Reset", "Shoot", "Ready"}."Shoot", s=w393, f=w394) -> (s? t:f=w395:enum16{"Reset", "Shoot", "Ready"})
              }
            }
          }
          frame "Bang Bang Control" {
            w404 = T20 0 items=["PercentOutput"=0, "Position"=1, "Velocity"=2, "Current"=3, "Follower"=5, "MotionProfile"=6, "MotionMagic"=7, "MotionProfileArc"=10, "Disabled"=15] ("Control Mode")
            n135 = case shown="\"Reset\"" w403 {
              selector: w403 -> [w406 w414 w423]
              tunnel: [w405 w413 w422] -> w402
              tunnel: w401 -> [_ _ w420]
              tunnel: [-1.0 ("Bang-Bang Cat Speed") 1.0 ("Bang-Bang Cat Speed") 0.0 ("Bang-Bang Cat Speed")] -> w400
              tunnel: w399 -> [w409 w416 _]
              tunnel: w398 -> [_ w415 _]
              frame "Reset" {
                n136 = Less?(x=w409, y=50) -> (x < y?=w410:bool)
                n137 = Select(t=enum16{"Reset", "Shoot", "Ready"}."Ready", s=w410, f=w406) -> (s? t:f=w405:enum16{"Reset", "Shoot", "Ready"})
              }
              frame "Shoot" {
                n138 = Greater?(x=w416, y=w415) -> (0:w417:bool)
                n139 = Select(t=enum16{"Reset", "Shoot", "Ready"}."Reset", s=w417, f=w414) -> (s? t:f=w413:enum16{"Reset", "Shoot", "Ready"})
              }
              frame "Ready", Default {
                n140 = Select(t=enum16{"Reset", "Shoot", "Ready"}."Shoot", s=w420, f=w423) -> (s? t:f=w422:enum16{"Reset", "Shoot", "Ready"})
              }
            }
          }
        }
      }
      frame "Puncher intake-shooter" {
        w427 = T20 0 items=["PercentOutput"=0, "Position"=1, "Velocity"=2, "Current"=3, "Follower"=5, "MotionProfile"=6, "MotionMagic"=7, "MotionProfileArc"=10, "Disabled"=15] ("Control Mode")
        w425 = T20 0 items=["PercentOutput"=0, "Position"=1, "Velocity"=2, "Current"=3, "Follower"=5, "MotionProfile"=6, "MotionMagic"=7, "MotionProfileArc"=10, "Disabled"=15] ("Control Mode")
      }
    }
    n141 = Divide(x=w251, y=4096) -> (x/y=w241:dbl)
    n142 = Divide(x=w241, y=3.141592653589793) -> (x/y=w237:dbl)
    n143 = Multiply(x=w237, y=180.0) -> (x*y=→"Mechanism Angle":dbl)
    n144 = call <vilib>:"CTRE_Phoenix_MotorControl_Set.vi"("Output"=w229, "Control Mode"=w230, "PhoenixMotorControlDevRef"=w231) -> ()  [unwired: 7 in, 2 out]
    n145 = call <vilib>:"CTRE_Phoenix_MotorControl_ConfigClosedLoopConstants.vi"("PhoenixMotorControlDevRef"=w250, "slotIdx"=0, "P"="P", "D"="D", "F"="F") -> ("PhoenixMotorControlDevRef"=w245:T9)  [unwired: 9 in, 1 out]
    n146 = Tick Count (ms)() -> (millisecond timer value=w272:u32)
    n147 = feedback #3() -> (w271:u32)  [unwired: 1 in]
    n148 = feedback-in #3(w272) -> ()
    n149 = Subtract(x=w272, y=w271) -> (x-y=→"Mechanism Loop Speed":u32)
    n150 = call <vilib>:"CTRE_Phoenix_MotorControl_ConfigMotionMagic.vi"("Acceleration"="Acceleration", "Cruise Velocity"="Cruise Velocity", "PhoenixMotorControlDevRef"=w245) -> ("PhoenixMotorControlDevRef"=w244:T9)  [unwired: 7 in, 1 out]
    n151 = call <vilib>:"CTRE_Phoenix_MotorControl_ConfigPeakOutput.vi"("Reverse Peak Percent Output"="Max Reset Speed", "Forward Peak Percent Output"="Max Shoot Speed", "PhoenixMotorControlDevRef"=w244) -> ("PhoenixMotorControlDevRef"=w249:T9)  [unwired: 7 in, 1 out]
    n152 = Wait (ms)(milliseconds to wait=u32 10) -> ()  [unwired: 1 out]
    n153 = call <vilib>:"CTRE_Phoenix_MotorControl_Set.vi"("Output"=w252, "Control Mode"=w253, "PhoenixMotorControlDevRef"=w249) -> ()  [unwired: 7 in, 2 out]
  }
  n154 = call <vilib>:"WPI_SolenoidRefNum Registry Get.vi"("refnum name"="Puncher 1") -> ("SolenoidDevRef"=w19:T22)  [unwired: 9 in, 1 out]
  n155 = call <vilib>:"WPI_SolenoidRefNum Registry Get.vi"("refnum name"="Puncher 2") -> ("SolenoidDevRef"=w16:T22)  [unwired: 9 in, 1 out]
  n156 = call <vilib>:"WPI_JoystickRefNum Registry Get.vi"("refnum name"="Joystick 2") -> ("JoystickDevRef"=w21:T5)  [unwired: 1 in, 9 out]
  n157 = call <vilib>:"WPI_CompressorRefNum Registry Get.vi"("refnum name"="Compressor") -> ("CompressorDevRef"=w18:T24)  [unwired: 9 in, 1 out]
  n158 = while {
    tunnel: w21 -> [w449]
    tunnel: w19 -> [w446]
    tunnel: w18 -> [w445]
    tunnel: w16 -> [w437]
    stop <- w433 stop-if-true
    # "Pneumatics"
    n159 = call <vilib>:"WPI_JoystickGetValues.vi"("JoystickDevRef"=w449) -> ("Buttons"=w447:bool[])  [unwired: 6 in, 4 out]
    n160 = call <vilib>:"WPI_CompressorGetEnableState.vi"("CompressorDevRef"=w445) -> ("error out"=w434:errorcluster, "Compressor Running"=→"C.Running":bool, "Enabled"=→"C.Monitoring":bool)  [unwired: 7 in, 1 out]
    n161 = Index Array(array=w447, index=7) -> (element=w436:bool)
    n162 = Unbundle By Name(w434) -> ("status"=w433:bool)
    n163 = Select(t=WPI_SolenoidValue."On" ("Value"), s=w436, f=WPI_SolenoidValue."Off" ("Value")) -> (s? t:f=w440:T25)
    n164 = Select(t=WPI_SolenoidValue."On" ("Value"), s=w436, f=WPI_SolenoidValue."Off" ("Value")) -> (s? t:f=w435:T25)
    n165 = call-poly <vilib>:"WPI_SolenoidSet.vi"("Value"=w440, "SolenoidDevRef"=w446) -> ()  [unwired: 8 in, 2 out]
    n166 = call-poly <vilib>:"WPI_SolenoidSet.vi"("Value"=w435, "SolenoidDevRef"=w437) -> ()  [unwired: 8 in, 2 out]
    n167 = Wait Until Next ms Multiple(millisecond multiple=u32 50) -> ()  [unwired: 1 out]
  }
